vi "Main.vi"   [LabVIEW 2015]
doc: "<b> </b> <b> </b>\n©2016 Q Software Innovations, LLC (QSI)\nwritten by Quentin Alldredge\nproduced in LabVIEW 2015"
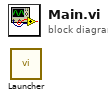
[diagram p0: block diagram]
diagram:
  n1 = call "Launcher.vi"() -> ()  [unwired: 12 in]
